vi "WPI_SimpleGyro_Reset.vi"(8 "error in":errorcluster, 10 "Reset? (T)":bool=TRUE, 11 "SimpleGyroDevRef":T1) -> (0 "error out":errorcluster, 3 "SimpleGyroDevRef":T1)   [LabVIEW 2014, in "SimpleGyro.lvlib"]
doc: "Resets the SimpleGyro zero position in software. This VI does NOT electrically reset the SimpleGyro."
uses:
  SimpleGyro.lvlib
  WPI_SimpleGyroDevRef.ctl
  <vilib>/Rock Robotics/SystemInterfaces/Typedef/FPGA_TypedefDigitalModule.ctl
  <vilib>/Rock Robotics/SystemInterfaces/spilib/spi_bus.ctl
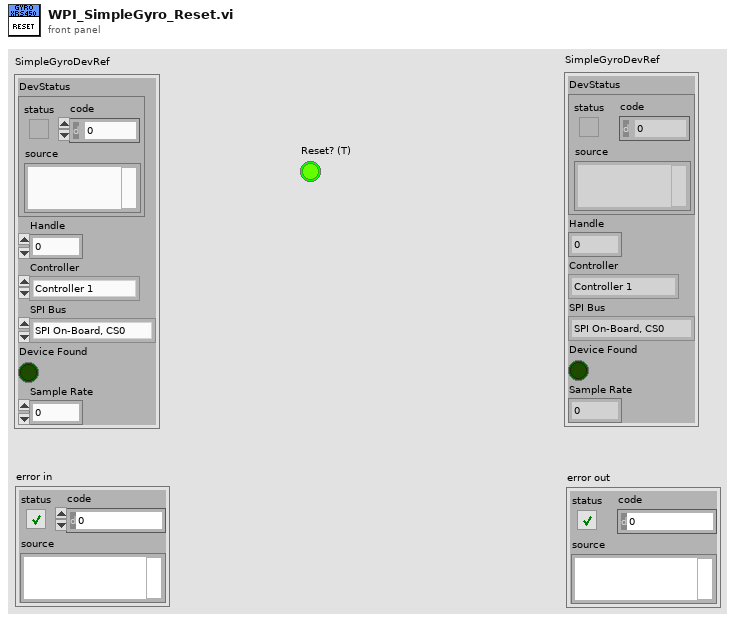
[diagram p1: front panel]
types:
  T1 = typedef "SimpleGyro.lvlib/WPI_SimpleGyroDevRef.ctl" = cluster{"DevStatus":errorcluster, "Handle":i32, "Controller":T2, "SPI Bus":T3, "Device Found":bool, "Sample Rate":dbl}
  T2 = typedef "FPGA_TypedefDigitalModule.ctl" = enum16{"Controller 1"}
  T3 = typedef "spi_bus.ctl" = enum16{"SPI On-Board, CS0", "SPI On-Board, CS1", "SPI On-Board, CS2", "SPI On-Board, CS3", "SPI MXP", "Invalid"}
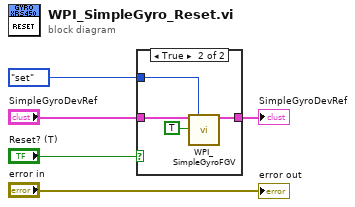
[diagram p0: block diagram]
diagram:
  n1 = case shown="True" "Reset? (T)" {
    tunnel: [w6 w10] -> w5
    tunnel: "SimpleGyroDevRef" -> [w6 w9]
    tunnel: enum16{"set", "get"}."set" ("Operation") -> [_ w8]
    frame False {
    }
    frame True {
      n2 = call "WPI_SimpleGyroFGV.vi"("SimpleGyroDevRef"=w9, "Operation"=w8, "Reset"=TRUE) -> ("SimpleGyroDevRef"=w10:T1)  [unwired: 8 in, 4 out]
    }
  }
  "SimpleGyroDevRef" <- w5
  "error out" <- "error in"
